vi "health_subpanel.vi"() -> ()   [LabVIEW 2018]
uses:
  health_state.ctl
  health_Loop_Clust.ctl
  ATA_RF_Acq/HDF5/HDF5_HealthData.ctl
  Epimedia_Connex_Source/Controls/Enums/LogLoopEnum.ctl
panel:
  in  "error in":errorcluster
  out "Hatch Command":bool
  in  "Sample Now":bool
  out "Faults Since":string
  out "Total Faults":i16
  out "Running LED":bool
  out "Progress Bar":dbl(slide) scale=0.0..60.0
  out "Error Dialog":string="Error Message Display Box"
  out "Values":dbl[](array[numeric]) format="%.3g"
  out "Faults":bool[](array[boolean])
  out "Units":string[](array[string])
  out "Label":string[](array[string])
  in  "Toggle Hatch":bool
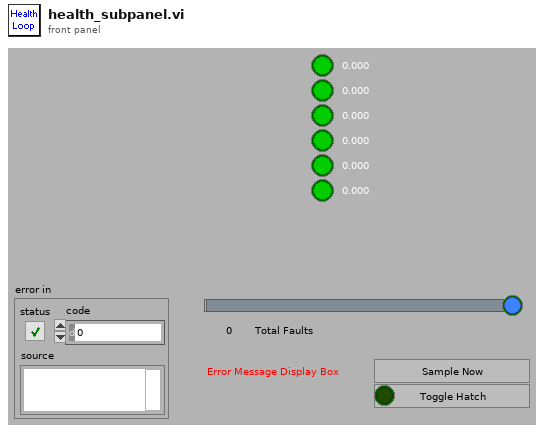
[diagram p1: front panel]
types:
  T1 = typedef "health_state.ctl" = enum16{"Health_Config", "Health_Wait", "Health_Read", "Health_Log", "Health_Exit"}
  T2 = typedef "health_Loop_Clust.ctl" = cluster{"nSignals":i32, "logname":string, "time":timestamp, "dir":path, "adamSerial":cluster{"port":refnum<visa-resource-name>, "timeout":u32, "baud":u32, "dataBits":u16, "stopBits":u16, "flowControl":u16, "parity":u16, "termChar":bool, "checkSum":bool}, "fiberSerial":cluster{"port1":refnum<visa-resource-name>, "port2":refnum<visa-resource-name>, "timeout":u32, "baud":u32, "dataBits":u16, "stopBits":u16, "flowControl":u16, "parity":u16, "termChar":bool, "checkSum":bool, "fiber1On":bool, "fiber2On":bool}, "signal":cluster{"src":enum16{"adam", "fiber", "te"}[], "id":string[], "ch":string[], "descrip":string[], "units":string[], "scale":dbl[], "hi":dbl[], "lo":dbl[], "rec":bool[], "fault":bool[], "val":dbl[]}, "teSerial":cluster{"port":refnum<visa-resource-name>, "timeout":u32, "baud":u32, "dataBits":u16, "stopBits":u16, "flowControl":u16, "parity":u16, "termChar":bool, "checkSum":bool, "checkSumVal":string}, "lograte":u32, "calSwitch":bool, "logoffset":dbl}
  T3 = typedef "HDF5_HealthData.ctl" = cluster{"Timestamp":dbl, "Time string":string, "Fault 1":bool, "Fault 2":bool, "Fault 3":bool, "Fault 4":bool, "Fault 5":bool, "Fault 6":bool, "Value 1":dbl, "Value 2":dbl, "Value 3":dbl, "Value 4":dbl, "Value 5":dbl, "Value 6":dbl}
  T4 = cluster{"port":refnum<visa-resource-name>, "timeout":u32, "baud":u32, "dataBits":u16, "stopBits":u16, "flowControl":u16, "parity":u16, "termChar":bool, "checkSum":bool}
  T5 = cluster{"port1":refnum<visa-resource-name>, "port2":refnum<visa-resource-name>, "timeout":u32, "baud":u32, "dataBits":u16, "stopBits":u16, "flowControl":u16, "parity":u16, "termChar":bool, "checkSum":bool, "fiber1On":bool, "fiber2On":bool}
  T6 = cluster{"port":refnum<visa-resource-name>, "timeout":u32, "baud":u32, "dataBits":u16, "stopBits":u16, "flowControl":u16, "parity":u16, "termChar":bool, "checkSum":bool, "checkSumVal":string}
  T7 = typedef "LogLoopEnum.ctl" = enum16{"Log_Init", "Log_Config", "Log_CfgAlarm", "Log_TimeDomain", "Log_Tone", "Log_NoiseTrace", "Log_NoiseSum", "Log_DO", "Log_AI", "Log_TC", "Log_Disdrom", "Log_Weather", "Log_TE", "Log_ADAM", "Log_UPS", "Log_ChkTime", "Log_Alarm", "Log_Write", "Log_Exit"}
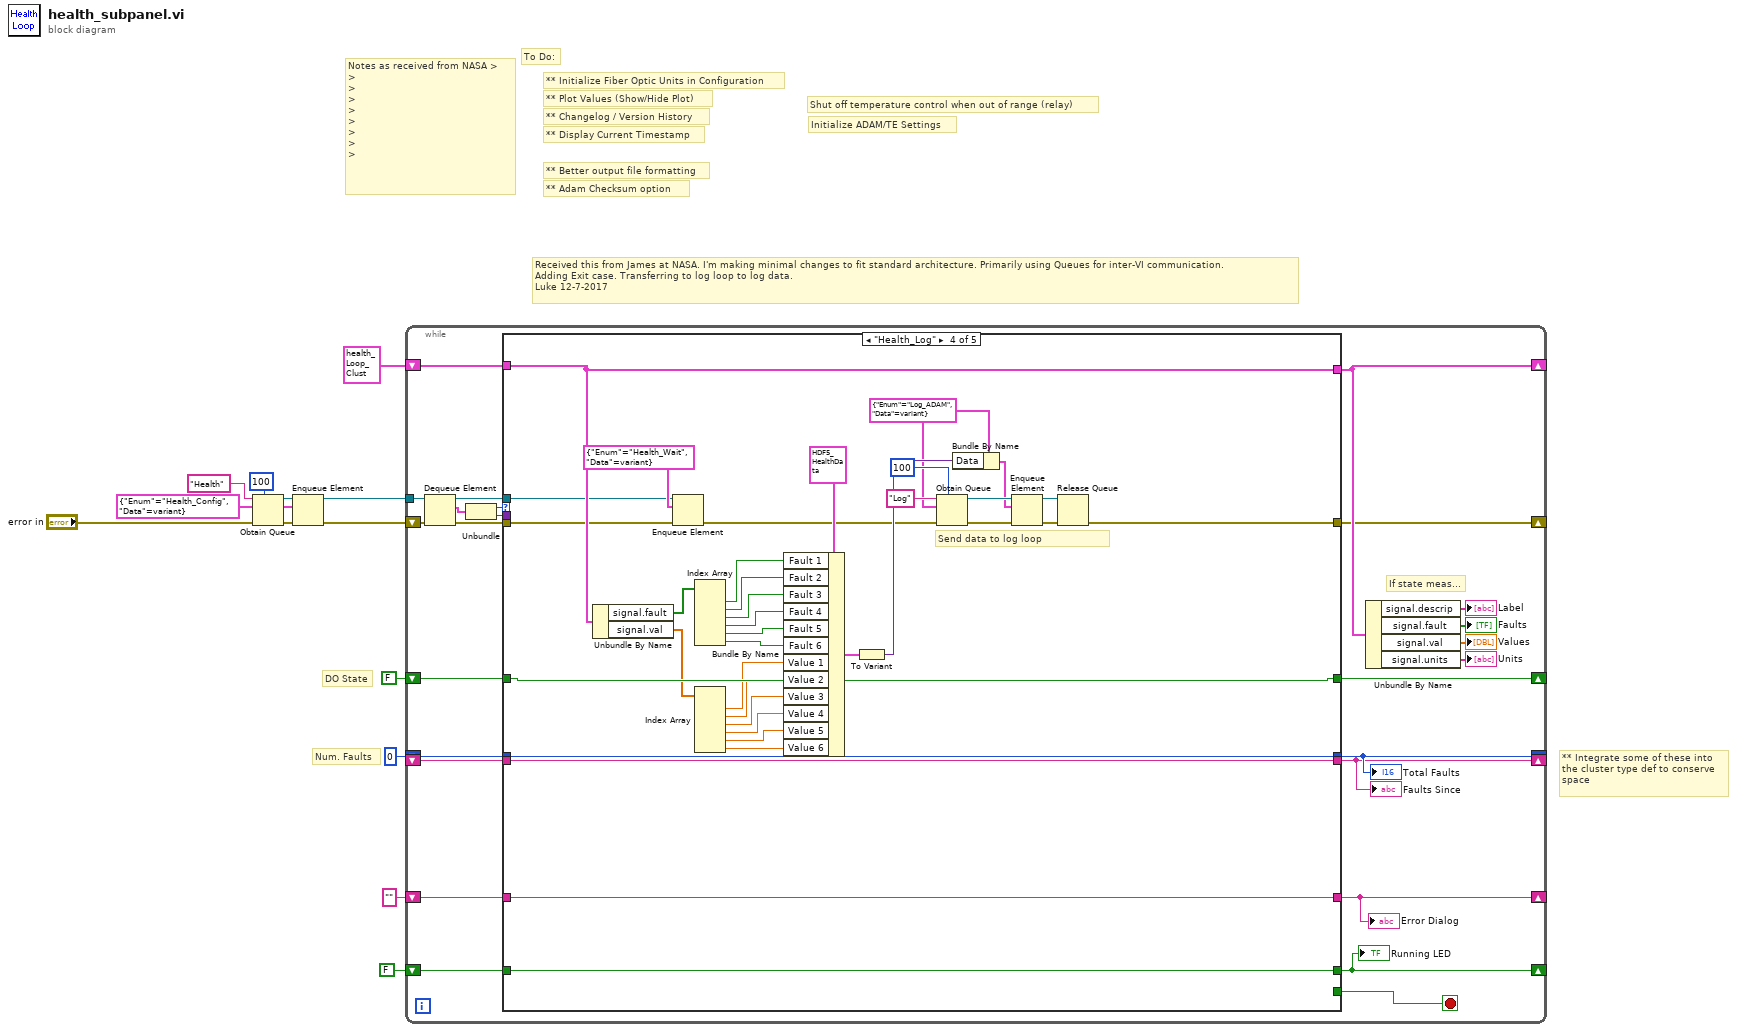
[diagram p0: block diagram]
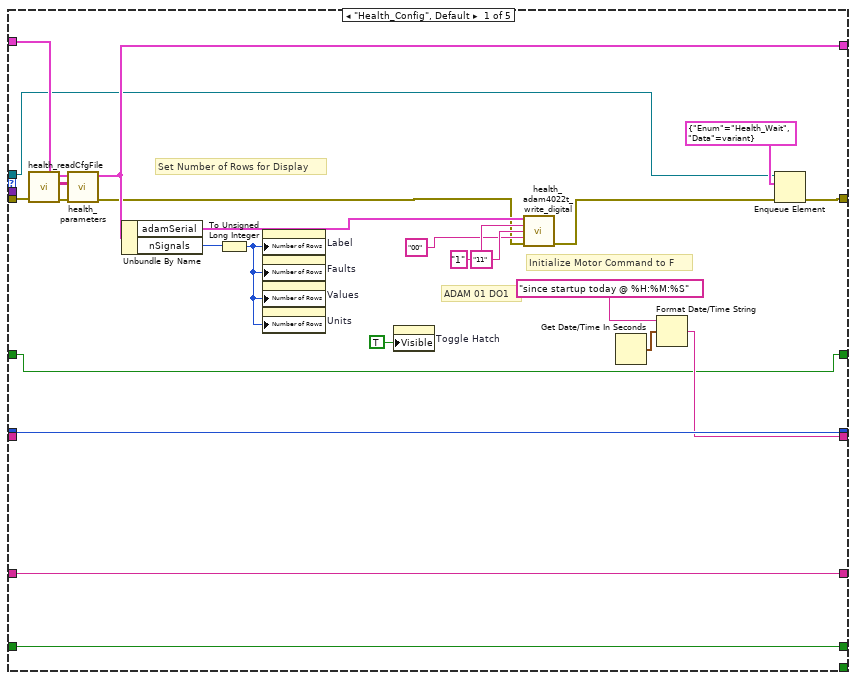
[diagram p2: hidden frame]
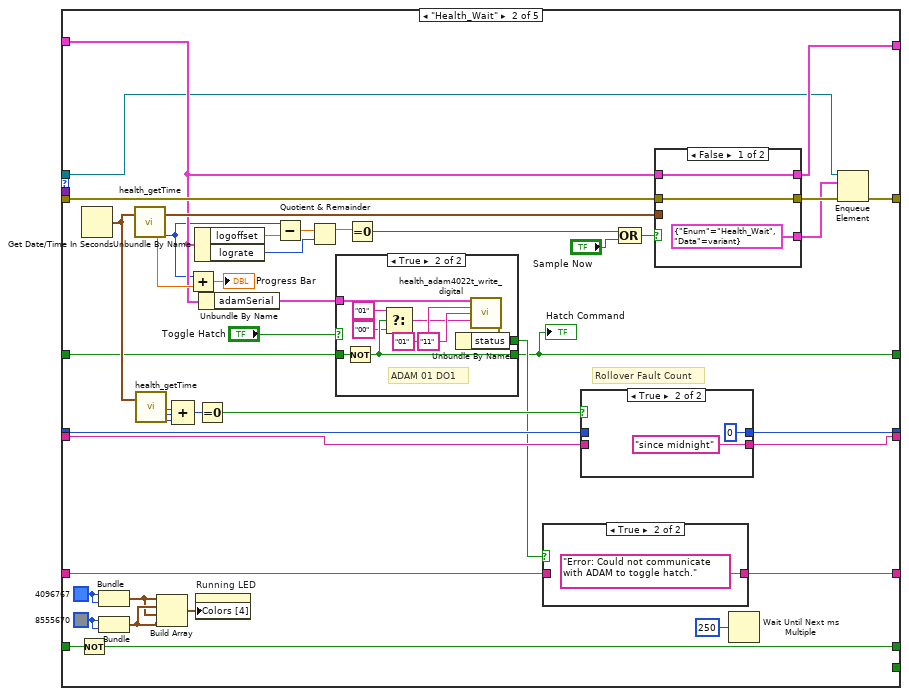
[diagram p3: hidden frame]
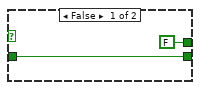
[diagram p5: hidden frame]
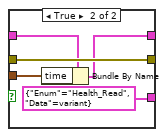
[diagram p7: hidden frame]
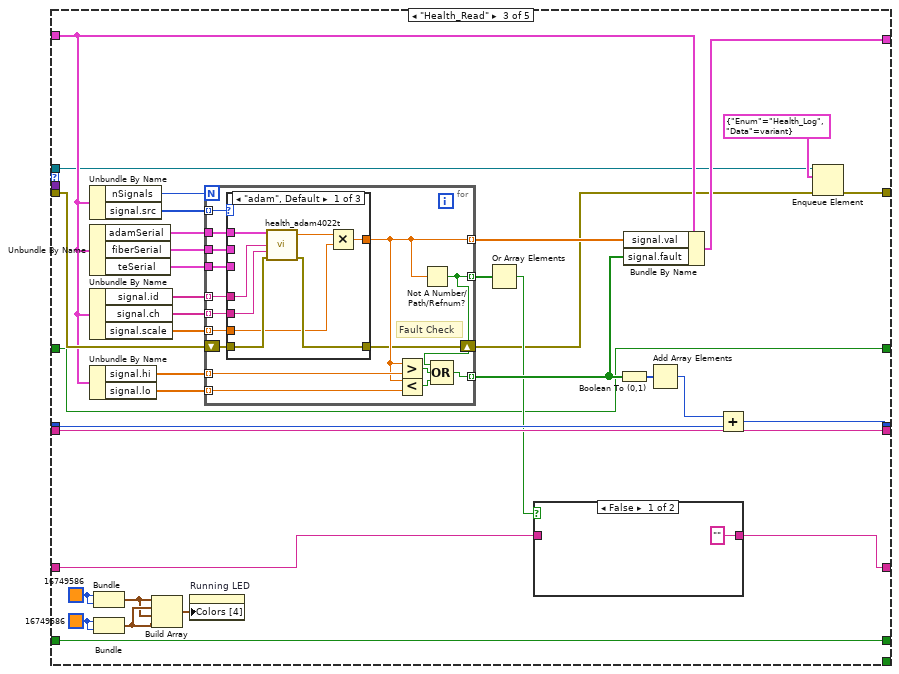
[diagram p8: hidden frame]
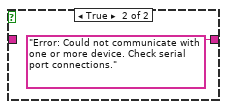
[diagram p9: hidden frame]
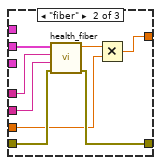
[diagram p10: hidden frame]
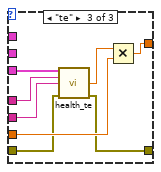
[diagram p11: hidden frame]
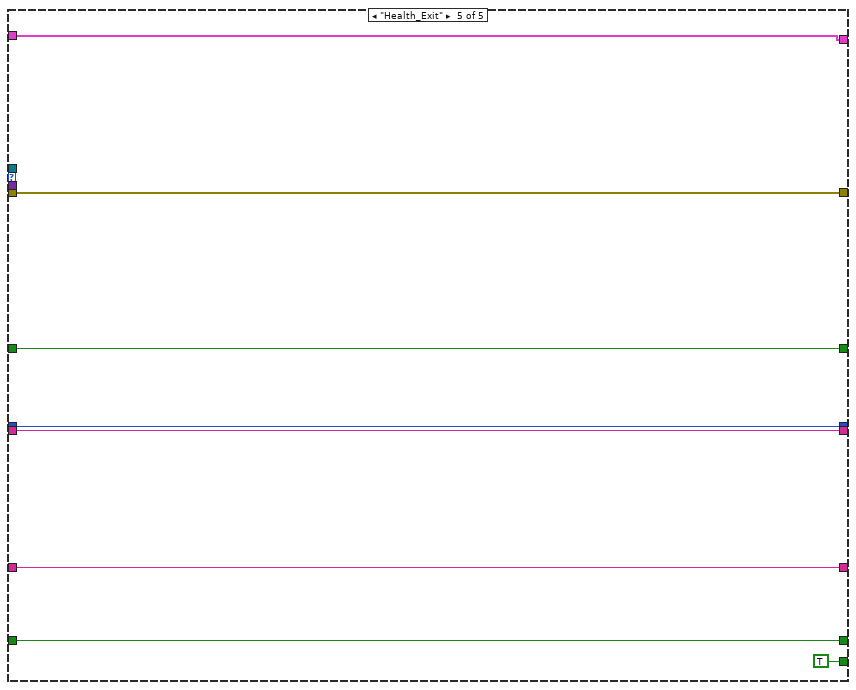
[diagram p12: hidden frame]
diagram:
  w4 = cluster{"Enum":T1, "Data":variant} {"Enum"=enum."Health_Config", "Data"=variant}
  # "Notes as received from NASA >\n>\n>\n>\n>\n>\n>\n>\n>"
  # "Received this from James at NASA. I'm making minimal changes to fit standard architecture. Primarily using Queues for inter-VI communication.\nAdding Exit case. Transferring to log loop to log data.\nLuke 12-7-2017"
  # "DO State"
  # "Initialize ADAM/TE Settings"
  # "Shut off temperature control when out of range (relay)"
  # "** Integrate some of these into\nthe cluster type def to conserve\nspace"
  # "** Changelog / Version History"
  # "** Plot Values (Show/Hide Plot)"
  # "** Display Current Timestamp"
  # "** Adam Checksum option"
  # "Num. Faults"
  # "** Better output file formatting"
  # "To Do:"
  # "** Initialize Fiber Optic Units in Configuration"
  n1 = Obtain Queue(max queue size (-1, unlimited)=100, name (unnamed)="Health", element data type=w4, error in (no error)="error in") -> (queue out=w6:refnum<queue>, error out=w5:errorcluster)  [unwired: 1 in, 1 out]
  n2 = Enqueue Element(queue=w6, element=w4, error in (no error)=w5) -> (queue out=w1:refnum<queue>, error out=w3:errorcluster)  [unwired: 1 in, 1 out]
  n3 = while {
    shift-right: [w34] -> _
    shift-left: T2 {"nSignals"=0, "logname"="", "time"=timestamp(0 s since 1904-01-01), "dir"=path "", "adamSerial"={"port"="", "timeout"=0, "baud"=0, "dataBits"=0, "stopBits"=0, "flowControl"=0, "parity"=0, "termChar"=FALSE, "checkSum"=FALSE}, "fiberSerial"={"port1"="", "port2"="", "timeout"=0, "baud"=0, "dataBits"=0, "stopBits"=0, "flowControl"=0, "parity"=0, "termChar"=FALSE, "checkSum"=FALSE, "fiber1On"=FALSE, "fiber2On"=FALSE}, "signal"={"src"=[], "id"=[], "ch"=[], "descrip"=[], "units"=[], "scale"=[], "hi"=[], "lo"=[], "rec"=[], "fault"=[], "val"=[]}, "teSerial"={"port"="", "timeout"=0, "baud"=0, "dataBits"=0, "stopBits"=0, "flowControl"=0, "parity"=0, "termChar"=FALSE, "checkSum"=FALSE, "checkSumVal"=""}, "lograte"=0, "calSwitch"=FALSE, "logoffset"=0.0} ("hDout") -> [w38]
    shift-right: [w24] -> _
    shift-left: w3 -> [w21]
    shift-right: [w36] -> _
    shift-left: FALSE -> [w37]
    shift-right: [w29] -> _
    shift-left: i16 0 -> [w30]
    shift-right: [w28] -> _
    shift-left: _ -> [w27]
    shift-right: [w26] -> _
    shift-left: "" ("Error Dialog") -> [w25]
    shift-right: [w23] -> _
    shift-left: FALSE -> [w22]
    tunnel: w1 -> [w19]
    stop <- w14 stop-if-true
    # "If state meas..."
    n4 = Dequeue Element(queue=w19, error in (no error)=w21) -> (queue out=w18:refnum<queue>, element=w17:cluster{"Enum":T1, "Data":variant}, error out=w20:errorcluster)  [unwired: 1 in, 1 out]
    n5 = Unbundle(w17) -> ("Enum"=w16:T1, "Data"=w15:variant)
    n6 = case shown="\"Health_Log\"" w16 {
      tunnel: w20 -> [w62 w92 w157 w236 w251]
      tunnel: [w57 w93 w158 w242 w250] -> w34
      tunnel: w38 -> [w59 w75 w142 w242 w250]
      tunnel: [w58 w101 w165 w243 w245] -> w36
      tunnel: w37 -> [w58 w102 w165 w243 w245]
      tunnel: [w55 w87 w149 w241 w248] -> w29
      tunnel: w30 -> [w55 w86 w148 w241 w248]
      tunnel: [w53 w85 w141 w240 w247] -> w28
      tunnel: w27 -> [_ w84 w141 w240 w247]
      tunnel: [w51 w73 w139 w239 w246] -> w26
      tunnel: w25 -> [w51 w72 w137 w239 w246]
      tunnel: [w40 w65 w134 w208 w251] -> w24
      tunnel: [w50 w67 w135 w238 w249] -> w23
      tunnel: w22 -> [w50 w76 w135 w238 w249]
      tunnel: w18 -> [w39 w64 w132 w235 _]
      tunnel: w15 -> [_ _ _ _ _]
      tunnel: [_ _ _ _ TRUE ("stop")] -> w14
      frame "Health_Config", Default {
        # "Initialize Motor Command to F"
        # "ADAM 01 DO1"
        # "Set Number of Rows for Display"
        n7 = call "health_readCfgFile.vi"("error in \n(no error)"=w62) -> ("error out"=w60:errorcluster, "parameters"=w61:string[][])  [unwired: 9 in]
        n8 = call "health_parameters.vi"("error in\n(no error)"=w60, "parameters"=w61, "hDin"=w59) -> ("error out"=w43:errorcluster, "hDout"=w57:T2)  [unwired: 7 in]
        n9 = Unbundle By Name(w57) -> ("adamSerial"=w47:T4, "nSignals"=w49:i32)
        n10 = To Unsigned Long Integer(number=w49) -> (unsigned 32bit integer=w56:u32)
        n11 = property on="Label" class="Arr (strict)"("Number of Rows"=w56) -> ()  [unwired: 2 in, 2 out]
        n12 = property on="Faults" class="Arr (strict)"("Number of Rows"=w56) -> ()  [unwired: 2 in, 2 out]
        n13 = property on="Values" class="Arr (strict)"("Number of Rows"=w56) -> ()  [unwired: 2 in, 2 out]
        n14 = property on="Units" class="Arr (strict)"("Number of Rows"=w56) -> ()  [unwired: 2 in, 2 out]
        n15 = property on="Toggle Hatch" class="Bool"("Visible"=TRUE) -> ()  [unwired: 2 in, 2 out]
        n16 = call "health_adam4022t_write_digital.vi"(0:w47, "Address"="1", "Channel"="11", "Value"="00" ("Address"), "Error In"=w43) -> ("Error Out"=w41:errorcluster)  [unwired: 8 in, 2 out]
        n17 = Get Date/Time In Seconds() -> (seconds since 1Jan1904=w52:timestamp)
        n18 = Format Date/Time String(time format string (%c)="since startup today @ %H:%M:%S", seconds (now)=w52) -> (date/time string=w53:string)  [unwired: 1 in]
        n19 = Enqueue Element(queue=w39, element=cluster{"Enum":T1, "Data":variant} {"Enum"=enum."Health_Wait", "Data"=variant}, error in (no error)=w41) -> (error out=w40:errorcluster)  [unwired: 1 in, 2 out]
      }
      frame "Health_Wait" {
        w99 = u32 8555670
        w98 = u32 4096767
        # "Rollover Fault Count"
        n20 = Not(x=w102) -> (.not. x?=w101:bool)
        n21 = Get Date/Time In Seconds() -> (seconds since 1Jan1904=w83:timestamp)
        n22 = Bundle(w98, w98) -> (w96:cluster{u32, u32})  [unwired: 1 in]
        n23 = Bundle(w99, w99) -> (w97:cluster{u32, u32})  [unwired: 1 in]
        n24 = call "health_getTime.vi"("Current Time"=w83) -> ("Fractional Seconds"=w95:dbl, "Seconds"=w70:u32)  [unwired: 11 in, 6 out]
        n25 = call "health_getTime.vi"("Current Time"=w83) -> ("Hour"=w89:u32, "Minutes"=w90:u32, "Seconds"=w91:u32)  [unwired: 11 in, 5 out]
        n26 = Build Array(w96, w97, w96, w97) -> (w100:cluster{u32, u32}[])
        n27 = Compound Arithmetic op=ADD(w89, w90, w91) -> (w103:u32)
        n28 = Add(x=w70, y=w95) -> (x+y=→"Progress Bar":dbl)
        n29 = Unbundle By Name(w75) -> ("logoffset"=w69:dbl, "lograte"=w81:u32)
        n30 = property on="Running LED" class="Bool (strict)"("Colors [4]"=w100) -> ()  [unwired: 2 in, 2 out]
        n31 = Equal To 0?(x=w103) -> (x = 0?=w88:bool)
        n32 = Unbundle By Name(w75) -> ("adamSerial"=w74:T4)
        n33 = Subtract(x=w70, y=w69) -> (x-y=w68:dbl)
        n34 = Quotient & Remainder(x=w68, y=w81) -> (x-y*floor(x/y)=w82:dbl)  [unwired: 1 out]
        n35 = case shown="True" "Toggle Hatch" {
          tunnel: [w108 w117] -> w67
          tunnel: w76 -> [w108 w118]
          tunnel: w74 -> [_ w115]
          tunnel: [FALSE ("status") w116] -> w71
          frame False {
          }
          frame True {
            # "ADAM 01 DO1"
            n36 = Not(x=w118) -> (.not. x?=w117:bool)
            n37 = Select(t="01" ("Address"), s=w117, f="00" ("Address")) -> (s? t:f=w109:string)
            n38 = call "health_adam4022t_write_digital.vi"(0:w115, "Address"="01", "Channel"="11", "Value"=w109) -> ("Error Out"=w112:errorcluster)  [unwired: 9 in, 2 out]
            n39 = Unbundle By Name(w112) -> ("status"=w116:bool)
          }
        }
        "Hatch Command" <- w67
        n40 = Equal To 0?(x=w82) -> (x = 0?=w80:bool)
        n41 = case shown="True" w71 {
          tunnel: [w105 "Error: Could not communicate with ADAM to toggle hatch." ("Error Dialog")] -> w73
          tunnel: w72 -> [w105 _]
          frame False {
          }
          frame True {
          }
        }
        n42 = case shown="True" w88 {
          tunnel: [w120 i16 0] -> w87
          tunnel: w86 -> [w120 _]
          tunnel: [w119 "since midnight" ("time format string (%c)")] -> w85
          tunnel: w84 -> [w119 _]
          frame False {
          }
          frame True {
          }
        }
        n43 = Compound Arithmetic op=OR(w80, "Sample Now") -> (w78:bool)
        n44 = case shown="False" w78 {
          tunnel: [cluster{"Enum":T1, "Data":variant} {"Enum"=enum."Health_Wait", "Data"=variant} cluster{"Enum":T1, "Data":variant} {"Enum"=enum."Health_Read", "Data"=variant}] -> w63
          tunnel: [w125 w127] -> w93
          tunnel: w75 -> [w125 w129]
          tunnel: [w124 w130] -> w66
          tunnel: w92 -> [w124 w130]
          tunnel: w83 -> [_ w128]
          frame False {
          }
          frame True {
            n45 = Bundle By Name(cluster=w129, "time"=w128) -> (w127:T2)
          }
        }
        n46 = Wait Until Next ms Multiple(millisecond multiple=u32 250 ("milliseconds to wait")) -> ()  [unwired: 1 out]
        n47 = Enqueue Element(queue=w64, element=w63, error in (no error)=w66) -> (error out=w65:errorcluster)  [unwired: 1 in, 2 out]
      }
      frame "Health_Read" {
        w164 = u32 16749586
        w163 = u32 16749586
        n48 = Unbundle By Name(w142) -> ("nSignals"=w159:i32, "signal.src"=w156:enum16{"adam", "fiber", "te"}[])
        n49 = Unbundle By Name(w142) -> ("adamSerial"=w147:T4, "fiberSerial"=w146:T5, "teSerial"=w136:T6)
        n50 = Unbundle By Name(w142) -> ("signal.id"=w145:string[], "signal.ch"=w144:string[], "signal.scale"=w143:dbl[])
        n51 = Unbundle By Name(w142) -> ("signal.hi"=w155:dbl[], "signal.lo"=w154:dbl[])
        n52 = Bundle(w163, w163) -> (w161:cluster{u32, u32})  [unwired: 1 in]
        n53 = Bundle(w164, w164) -> (w162:cluster{u32, u32})  [unwired: 1 in]
        n54 = Build Array(w161, w162, w161, w162) -> (w160:cluster{u32, u32}[])
        n55 = property on="Running LED" class="Bool (strict)"("Colors [4]"=w160) -> ()  [unwired: 2 in, 2 out]
        n56 = for {
          N: w159 -> [_]
          tunnel: w145 -> [w183] mode=indexing
          tunnel: w144 -> [w182] mode=indexing
          tunnel: [w171] -> w153 mode=indexing
          tunnel: w155 -> [w181] mode=indexing
          tunnel: w154 -> [w180] mode=indexing
          tunnel: w156 -> [w179] mode=indexing
          tunnel: [w176] -> w152 mode=indexing
          tunnel: w143 -> [w174] mode=indexing
          tunnel: w147 -> [w173]
          tunnel: w146 -> [w172]
          tunnel: [w169] -> w140 mode=indexing
          tunnel: w136 -> [w170]
          shift-right: [w168] -> w131
          shift-left: w157 -> [w175]
          # "Fault Check"
          n57 = case shown="\"adam\", Default" w179 {
            tunnel: w183 -> [w191 w196 w204]
            tunnel: w182 -> [w190 w195 w201]
            tunnel: [w185 w197 w206] -> w171
            tunnel: w175 -> [w189 w199 w203]
            tunnel: [w188 w198 w202] -> w168
            tunnel: w174 -> [w186 w192 w207]
            tunnel: w173 -> [w184 _ _]
            tunnel: w172 -> [_ w194 _]
            tunnel: w170 -> [_ _ w205]
            frame "adam", Default {
              n58 = call "health_adam4022t.vi"(0:w184, "Address"=w191, "Channel"=w190, "Error In"=w189) -> ("Value"=w187:dbl, "Error Out"=w188:errorcluster)  [unwired: 10 in]
              n59 = Multiply(x=w187, y=w186) -> (x*y=w185:dbl)
            }
            frame "fiber" {
              n60 = call "health_fiber.vi"("fiberSerial"=w194, "Address"=w196, "Channel"=w195, "Error In"=w199) -> ("Value"=w193:dbl, "Error Out"=w198:errorcluster)  [unwired: 4 in, 1 out]
              n61 = Multiply(x=w193, y=w192) -> (x*y=w197:dbl)
            }
            frame "te" {
              n62 = call "health_te.vi"("teSerial"=w205, "Hex Address"=w204, "Command"=w201, "Error In"=w203) -> ("Response"=w200:dbl, "error out"=w202:errorcluster)  [unwired: 8 in, 2 out]
              n63 = Multiply(x=w200, y=w207) -> (x*y=w206:dbl)
            }
          }
          n64 = Greater?(x=w171, y=w181) -> (0:w178:bool)
          n65 = Less?(x=w171, y=w180) -> (x < y?=w177:bool)
          n66 = Not A Number/Path/Refnum?(number/path/refnum=w171) -> (NaN/Path/Refnum?=w169:bool)
          n67 = Compound Arithmetic op=OR(w169, w178, w177) -> (w176:bool)
        }
        n68 = Or Array Elements(Boolean array=w140) -> (logical OR=w138:bool)
        n69 = case shown="False" w138 {
          tunnel: ["" ("Error Dialog") "Error: Could not communicate with one or more device. Check serial port connections." ("Error Dialog")] -> w139
          tunnel: w137 -> [_ _]
          frame False {
          }
          frame True {
          }
        }
        n70 = Boolean To (0,1)(Boolean=w152) -> (0, 1=w150:i16[])
        n71 = Bundle By Name(cluster=w142, "signal.val"=w153, "signal.fault"=w152) -> (w158:T2)
        n72 = Add Array Elements(numeric array=w150) -> (sum=w151:i16)
        n73 = Add(x=w151, y=w148) -> (x+y=w149:i16)
        n74 = Enqueue Element(queue=w132, element=cluster{"Enum":T1, "Data":variant} {"Enum"=enum."Health_Log", "Data"=variant}, error in (no error)=w131) -> (error out=w134:errorcluster)  [unwired: 1 in, 2 out]
      }
      frame "Health_Log" {
        w210 = cluster{"Enum":T7, "Data":variant} {"Enum"=enum."Log_ADAM", "Data"=variant}
        # "Send data to log loop"
        n75 = Unbundle By Name(w242) -> ("signal.fault"=w232:bool[], "signal.val"=w234:dbl[])
        n76 = Enqueue Element(queue=w235, element=cluster{"Enum":T1, "Data":variant} {"Enum"=enum."Health_Wait", "Data"=variant}, error in (no error)=w236) -> (error out=w209:errorcluster)  [unwired: 1 in, 2 out]
        n77 = Index Array(array=w232) -> (element #1=w231:bool, element #2=w230:bool, element #3=w229:bool, element #4=w228:bool, element #5=w227:bool, element #6=w226:bool)  [unwired: 6 in]
        n78 = Index Array(array=w234) -> (element #1=w225:dbl, element #2=w224:dbl, element #3=w223:dbl, element #4=w222:dbl, element #5=w221:dbl, element #6=w220:dbl)  [unwired: 6 in]
        n79 = Bundle By Name(cluster=T3 {"Timestamp"=0.0, "Time string"="", "Fault 1"=FALSE, "Fault 2"=FALSE, "Fault 3"=FALSE, "Fault 4"=FALSE, "Fault 5"=FALSE, "Fault 6"=FALSE, "Value 1"=0.0, "Value 2"=0.0, "Value 3"=0.0, "Value 4"=0.0, "Value 5"=0.0, "Value 6"=0.0}, "Fault 1"=w231, "Fault 2"=w230, "Fault 3"=w229, "Fault 4"=w228, "Fault 5"=w227, "Fault 6"=w226, "Value 1"=w225, "Value 2"=w224, "Value 3"=w223, "Value 4"=w222, "Value 5"=w221, "Value 6"=w220) -> (w212:T3)
        n80 = To Variant(anything=w212) -> (Variant=w211:variant)
        n81 = Obtain Queue(max queue size (-1, unlimited)=100, name (unnamed)="Log", element data type=w210, error in (no error)=w209) -> (queue out=w217:refnum<queue>, error out=w216:errorcluster)  [unwired: 1 in, 1 out]
        n82 = Bundle By Name(cluster=w210, "Data"=w211) -> (w215:cluster{"Enum":T7, "Data":variant})
        n83 = Enqueue Element(queue=w217, element=w215, error in (no error)=w216) -> (queue out=w214:refnum<queue>, error out=w213:errorcluster)  [unwired: 1 in, 1 out]
        n84 = Release Queue(queue=w214, error in (no error)=w213) -> (error out=w208:errorcluster)  [unwired: 1 in, 2 out]
      }
      frame "Health_Exit" {
      }
    }
    "Running LED" <- w36
    "Total Faults" <- w29
    "Faults Since" <- w28
    "Error Dialog" <- w26
    n85 = Unbundle By Name(w34) -> ("signal.descrip"=→"Label":string[], "signal.fault"=→"Faults":bool[], "signal.val"=→"Values":dbl[], "signal.units"=→"Units":string[])
  }
